vi "[TN#5] FRA example (A).vi"() -> ()   [LabVIEW 2012]
uses:
  C:/Program Files/Metrohm Autolab/Autolab SDK 1.10/EcoChemie.Autolab.Sdk.dll
  EcoChemie.Autolab.Sdk.dll
panel:
  out "-Phase":dbl[](array[numeric])
  out "Frequency":dbl[](array[numeric])
  out "-Z''":dbl[](array[numeric])
  out "Z'":dbl[](array[numeric])
  out "Z":dbl[](array[numeric])
  in  "load":bool
  out "Blacklisted Commands detected":bool
  out "Bode phase":cluster{"Y":dbl[], "Y":dbl[]}[](graph)
  out "E & I":cluster{"Y":dbl[], "Y":dbl[]}[](graph)
  in  "Save":bool
  in  "Save data as .nox (Path + filename.nox)":string
  in  "Hardware Setup File":path
  in  "Embedded Exe File":path
  in  "Load Procedure":path
  out "Nyquist":cluster{"Y":dbl[], "Y":dbl[]}[](graph)
  out "Bode Z":cluster{"Y":dbl[], "Y":dbl[]}[](graph)
  out "Measurement active":bool
  in  "abort":bool
  in  "stop":bool
  in  "Start Measure":bool
  out "Autolab Connected":bool
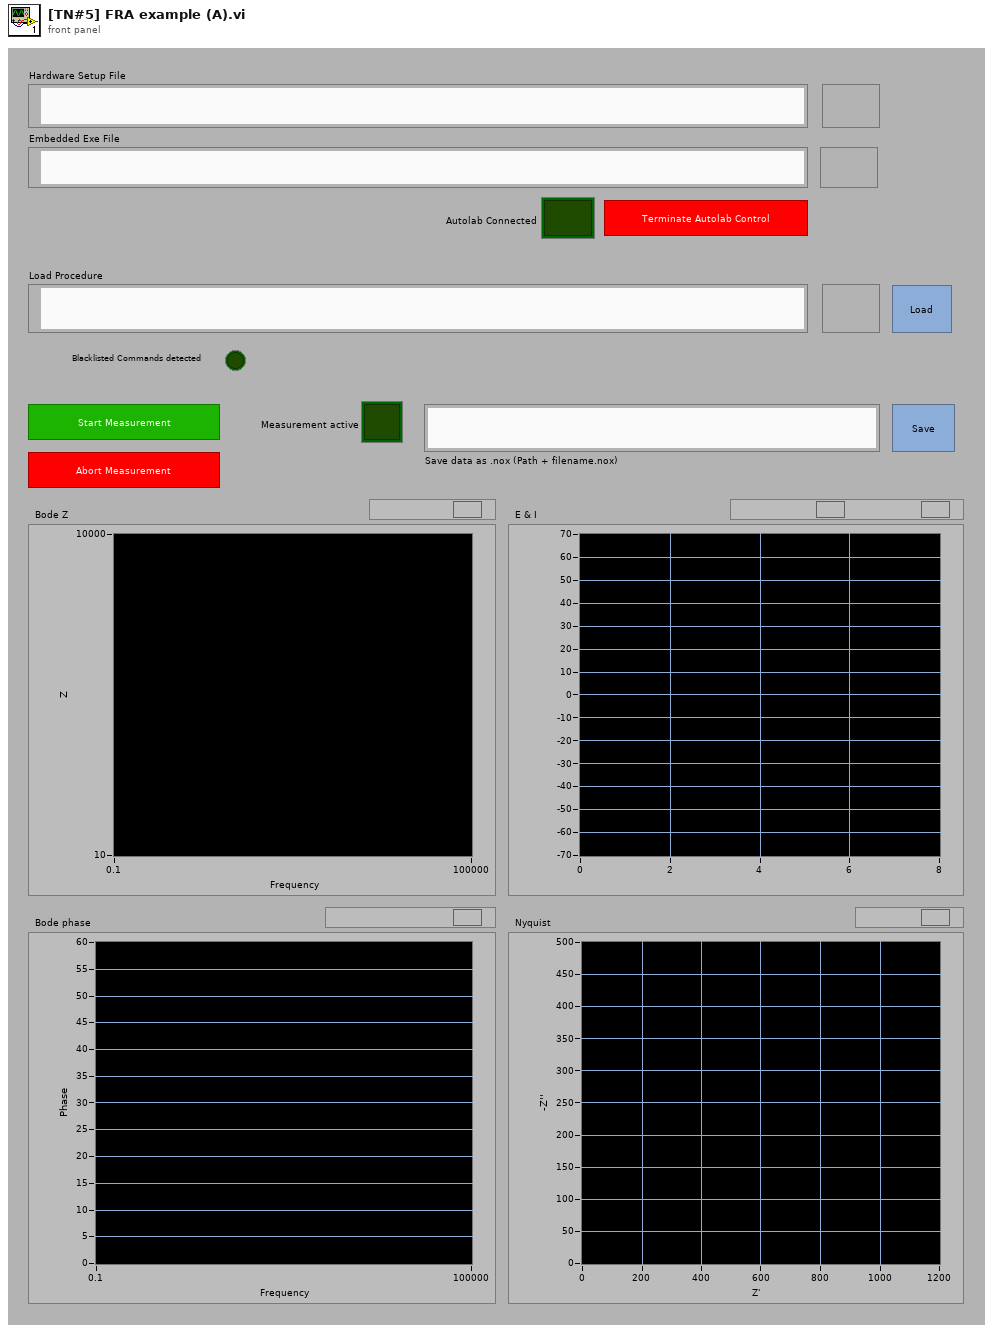
[diagram p1: front panel]
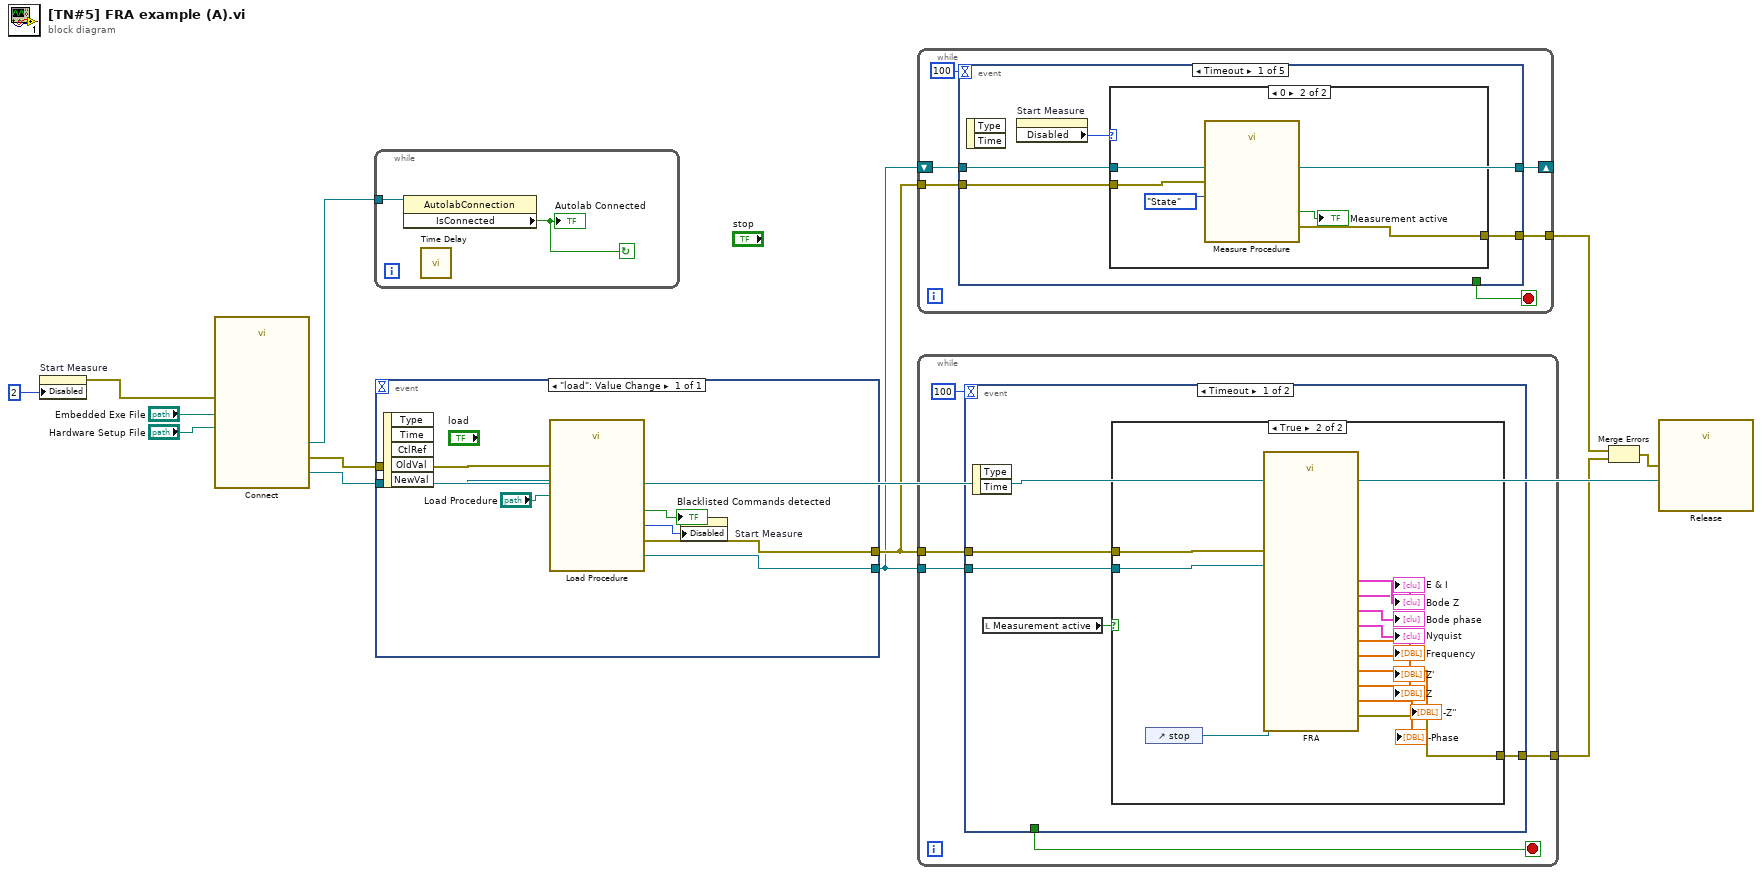
[diagram p0: block diagram]
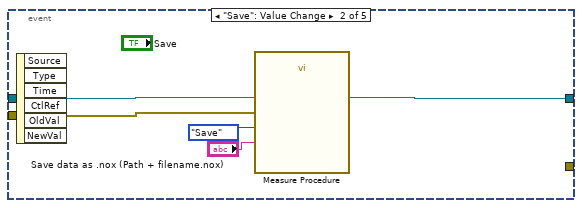
[diagram p3: hidden frame]
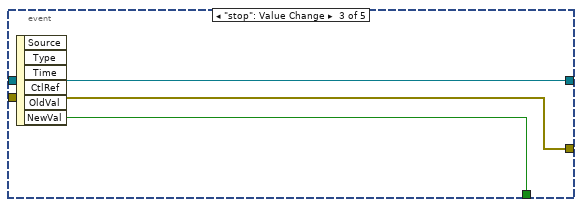
[diagram p4: hidden frame]
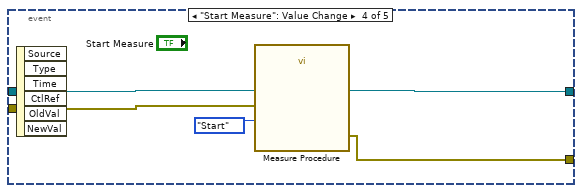
[diagram p5: hidden frame]
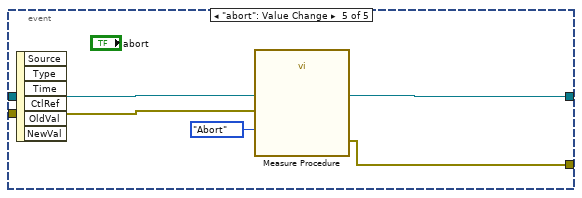
[diagram p6: hidden frame]
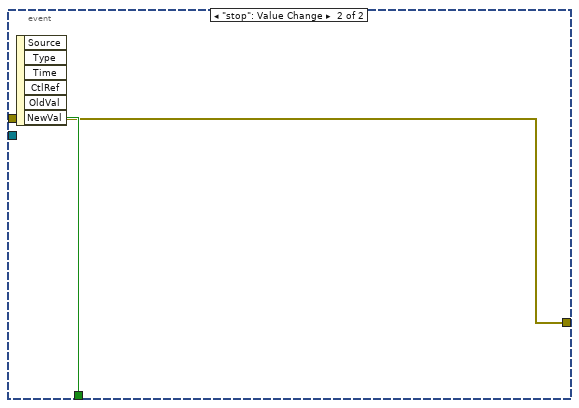
[diagram p8: hidden frame]
diagram:
  n1 = property on="Start Measure" class="Bool"("Disabled"=u8 2) -> (error out=w9:errorcluster)  [unwired: 2 in, 1 out]
  n2 = call "Connect.vi"("Embedded Exe File"="Embedded Exe File", "Hardware Setup File"="Hardware Setup File", "error in (no error)"=w9) -> ("AutolabConnection"=w12:refnum<k24>, "instrument"=w6:refnum<k24>, "error out"=w7:errorcluster)  [unwired: 10 out]
  n3 = while {
    tunnel: w12 -> [w13]
    stop <- w14 continue-if-true
    n4 = property class="AutolabConnection"(reference=w13) -> ("IsConnected"=w14:bool)  [unwired: 1 in, 2 out]
    "Autolab Connected" <- w14
    n5 = call "Time Delay"() -> ()  [unwired: 2 in, 10 out]
  }
  n6 = event shown="[0] \"load\": Value Change" {
    selector: _ -> [_]
    dyn-events: _ -> [_]
    timeout: _ -> [_]
    tunnel: w7 -> [w21]
    tunnel: w6 -> [w20]
    tunnel: [w15] -> w2
    tunnel: [w16] -> w5
    event "load": Value Change {
      n7 = event-data() -> ()  [unwired: 6 out]
      n8 = call "Load Procedure.vi"("error in (no error)"=w21, "Procedure"="Load Procedure", "Instrument"=w20) -> ("error out"=w16:errorcluster, "Contains"=→"Blacklisted Commands detected":bool, "Numeric"=w17:i32, "LoadProcedure"=w15:refnum<k24>)  [unwired: 5 out]
      n9 = property on="Start Measure" class="Bool"("Disabled"=w17) -> ()  [unwired: 2 in, 2 out]
    }
  }
  n10 = while {
    tunnel: w5 -> [w25]
    tunnel: [w24] -> w4
    shift-right: [w22] -> _
    shift-left: w2 -> [w23]
    stop <- w26 stop-if-true
    n11 = event shown="[0] Timeout" {
      selector: _ -> [_ _ _ _ _]
      dyn-events: _ -> [_ _ _ _ _]
      timeout: 100 -> [_ _ _ _ _]
      tunnel: [_ _ w44 _ _] -> w26
      tunnel: w25 -> [w30 w38 w42 w47 w51]
      tunnel: w23 -> [w28 w39 w43 w45 w49]
      tunnel: [w29 _ w42 w46 w50] -> w24
      tunnel: [w28 w39 w43 w45 w49] -> w22
      event Timeout {
        n12 = event-data() -> ()  [unwired: 3 out]
        n13 = property on="Start Measure" class="Bool"() -> ("Disabled"=w31:u8)  [unwired: 2 in, 2 out]
        n14 = case shown="0" w31 {
          tunnel: w30 -> [w32 w35]
          tunnel: w28 -> [_ w34]
          tunnel: [w32 w33] -> w29
          frame 2, Default {
          }
          frame 0 {
            n15 = call "Measure Procedure.vi"("error in"=w35, "Request for procedure"=enum16{"State", "Save", "Abort", "Start"}."State", "LoadProcedure"=w34) -> ("error out"=w33:errorcluster, "IsMeasuring"=→"Measurement active":bool)  [unwired: 1 in, 6 out]
          }
        }
      }
      event "Save": Value Change {
        n16 = event-data() -> ()  [unwired: 7 out]
        n17 = call "Measure Procedure.vi"("error in"=w38, "fileName"="Save data as .nox (Path + filename.nox)", "Request for procedure"=enum16{"State", "Save", "Abort", "Start"}."Save", "LoadProcedure"=w39) -> ()  [unwired: 8 out]
      }
      event "stop": Value Change {
        n18 = event-data() -> ("NewVal"=w44:bool)  [unwired: 6 out]
      }
      event "Start Measure": Value Change {
        n19 = event-data() -> ()  [unwired: 7 out]
        n20 = call "Measure Procedure.vi"("error in"=w47, "Request for procedure"=enum16{"State", "Save", "Abort", "Start"}."Start", "LoadProcedure"=w45) -> ("error out"=w46:errorcluster)  [unwired: 1 in, 7 out]
      }
      event "abort": Value Change {
        n21 = event-data() -> ()  [unwired: 7 out]
        n22 = call "Measure Procedure.vi"("error in"=w51, "Request for procedure"=enum16{"State", "Save", "Abort", "Start"}."Abort", "LoadProcedure"=w49) -> ("error out"=w50:errorcluster)  [unwired: 1 in, 7 out]
      }
    }
  }
  n23 = while {
    tunnel: w2 -> [w57]
    tunnel: w5 -> [w56]
    tunnel: [w54] -> w3
    stop <- w55 stop-if-true
    n24 = event shown="[0] Timeout" {
      selector: _ -> [_ _]
      dyn-events: _ -> [_ _]
      timeout: 100 -> [_ _]
      tunnel: w57 -> [w61 _]
      tunnel: w56 -> [w60 w76]
      tunnel: [_ w77] -> w55
      tunnel: [w58 w76] -> w54
      event Timeout {
        n25 = event-data() -> ()  [unwired: 3 out]
        n26 = local read "Measurement active"() -> (w59:bool)
        n27 = case shown="True" w59 {
          tunnel: w61 -> [_ w71]
          tunnel: w60 -> [w62 w70]
          tunnel: [w62 w69] -> w58
          frame False {
          }
          frame True {
            n28 = control-ref of="stop"() -> (w72:refnum<vi>)
            n29 = call "FRA.vi"("LoadProcedure"=w71, "stop"=w72, "error in"=w70) -> ("Bode phase"=→"Bode phase":cluster{"Y":dbl[], "Y":dbl[]}[], "Bode Z"=→"Bode Z":cluster{"Y":dbl[], "Y":dbl[]}[], "Nyquist"=→"Nyquist":cluster{"Y":dbl[], "Y":dbl[]}[], "E & I"=→"E & I":cluster{"Y":dbl[], "Y":dbl[]}[], "-Phase"=→"-Phase":dbl[], "Frequency"=→"Frequency":dbl[], "-Z''"=→"-Z''":dbl[], "Z"=→"Z":dbl[], "Z'"=→"Z'":dbl[], "error out"=w69:errorcluster)  [unwired: 15 out]
          }
        }
      }
      event "stop": Value Change {
        n30 = event-data() -> ("NewVal"=w77:bool)  [unwired: 6 out]
      }
    }
  }
  n31 = Merge Errors(w4, w3) -> (w1:errorcluster)
  n32 = call "Release.vi"("error in (no error)"=w1, "Instrument"=w6) -> ()  [unwired: 1 in, 9 out]
